vi "prompt user for configuration.vi"(8 "error in (no error)":errorcluster) -> (0 "error out":errorcluster, 2 "cancelled":bool, 3 "selected path":path)   [LabVIEW 2017, in "Data Sharing Framework System Explorer.lvlib"]
uses:
  Data Sharing Framework System Explorer.lvlib
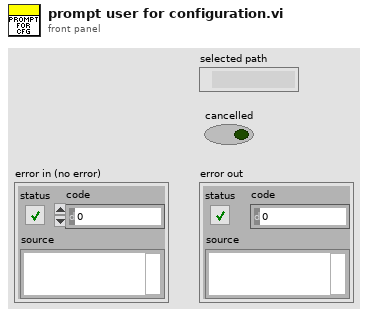
[diagram p1: front panel]
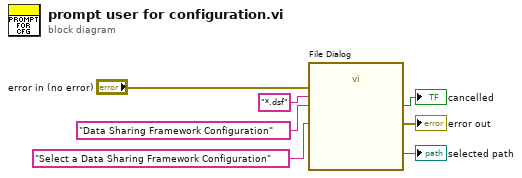
[diagram p0: block diagram]
diagram:
  n1 = call "File Dialog"("prompt"="Select a Data Sharing Framework Configuration", "error in"="error in (no error)", "pattern (all files)"="*.dsf", "pattern label"="Data Sharing Framework Configuration") -> ("selected path"=→"selected path":path, "cancelled"=→"cancelled":bool, "error out"=→"error out":errorcluster)  [unwired: 8 in, 1 out]
